vi "TIFF-Close Stack.vi"(0 "stack in":T1={"file"=refnum, "IFD"=[], "offset"=0, "byte order"=enum."little-endian", "image size"=0, "IFD size"=0, "max frames"=0, "frames"=0}, 11 "error in":errorcluster) -> (4 "stack out":T1={"file"=refnum, "IFD"=[], "offset"=0, "byte order"=enum."little-endian", "image size"=0, "IFD size"=0, "max frames"=0, "frames"=0}, 15 "error out":errorcluster)   [LabVIEW 2020]
uses:
  TIFF-Write State.ctl
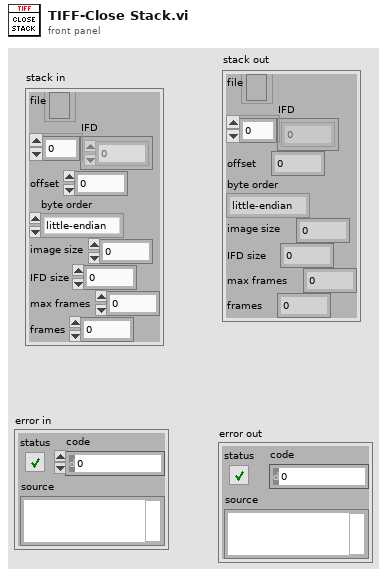
[diagram p1: front panel]
types:
  T1 = typedef "TIFF-Write State.ctl" = cluster{"file":refnum<file>, "IFD":u8[], "offset":u32, "byte order":enum16{"big-endian, network order", "native, host order", "little-endian"}, "image size":u32, "IFD size":u32, "max frames":u32, "frames":u32}
  T2 = enum16{"big-endian, network order", "native, host order", "little-endian"}
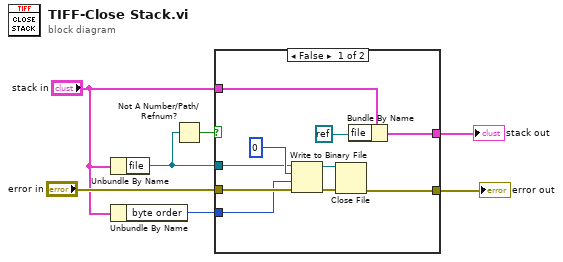
[diagram p0: block diagram]
diagram:
  n1 = Unbundle By Name("stack in") -> ("file"=w2:refnum<file>)
  n2 = Unbundle By Name("stack in") -> ("byte order"=w3:T2)
  n3 = Not A Number/Path/Refnum?(number/path/refnum=w2) -> (NaN/Path/Refnum?=w1:bool)
  n4 = case shown="False" w1 {
    tunnel: [w17 w19] -> w7
    tunnel: [w16 w18] -> w6
    tunnel: w2 -> [w12 _]
    tunnel: "error in" -> [w11 w18]
    tunnel: "stack in" -> [w10 w19]
    tunnel: w3 -> [w9 _]
    frame False {
      n5 = Write to Binary File(file (use dialog)=w12, data=u32 0, error in=w11, 9:w9) -> (refnum out=w13:refnum<file>, error out=w8:errorcluster)  [unwired: 2 in, 1 out]
      n6 = Close File(refnum=w13, error in=w8) -> (error out=w16:errorcluster)  [unwired: 1 out]
      n7 = Bundle By Name(cluster=w10, "file"=refnum<k0> refnum) -> (w17:T1)
    }
    frame True {
    }
  }
  "stack out" <- w7
  "error out" <- w6
